vi "fgv_Abort Acq and Logging.vi"(8 "error in (no error)":errorcluster, 9 "Function":T1, 11 "Live Imaging?":bool) -> (0 "error out":errorcluster, 3 "Abort acquisition":bool)   [LabVIEW 2013]
uses:
  Typedefs/Read Write Enum.ctl
  General Globals.vi
panel:
  # "SUBROUTINE"
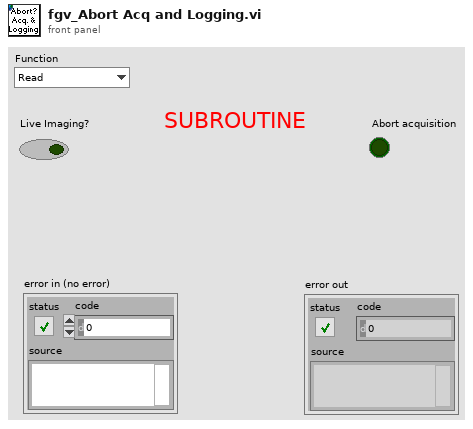
[diagram p1: front panel]
types:
  T1 = typedef "Read Write Enum.ctl" = enum16{"Read", "Write"}
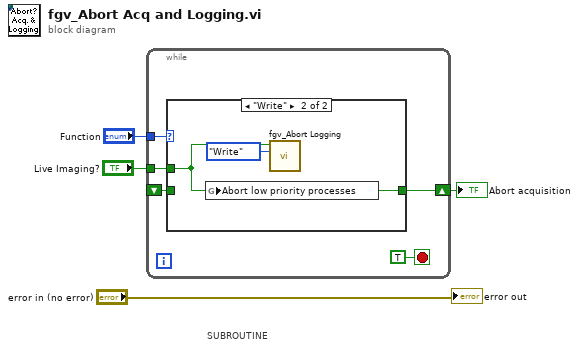
[diagram p0: block diagram]
diagram:
  # "SUBROUTINE"
  n1 = while {
    tunnel: "Function" -> [w8]
    tunnel: "Live Imaging?" -> [w7]
    shift-right: [w6] -> w2
    shift-left: _ -> [w5]
    stop <- TRUE stop-if-true
    n2 = case shown="\"Write\"" w8 {
      tunnel: w7 -> [_ w11]
      tunnel: [w10 w11] -> w6
      tunnel: w5 -> [w10 _]
      frame "Read", Default {
      }
      frame "Write" {
        n3 = global write "General Globals.vi" "Abort low priority processes"(w11) -> ()
        n4 = call "fgv_Abort Logging.vi"("Function"=Read_Write_Enum."Write", "Live Imaging?"=w11) -> ()  [unwired: 8 in, 2 out]
      }
    }
  }
  "Abort acquisition" <- w2
  "error out" <- "error in (no error)"
